vi "GetSingleAnalogInputVal.vi"(8 "error in (no error)":errorcluster, 11 "SerialPortRef":T1) -> (0 "error out":errorcluster, 1 "Scaled Voltage":dbl, 2 "Raw Voltage":u32, 3 "SerialPortRef 2":T1)   [LabVIEW 2015]
uses:
  <vilib>/Rock Robotics/WPI/SerialPort/WPI_SerialPortRef.ctl
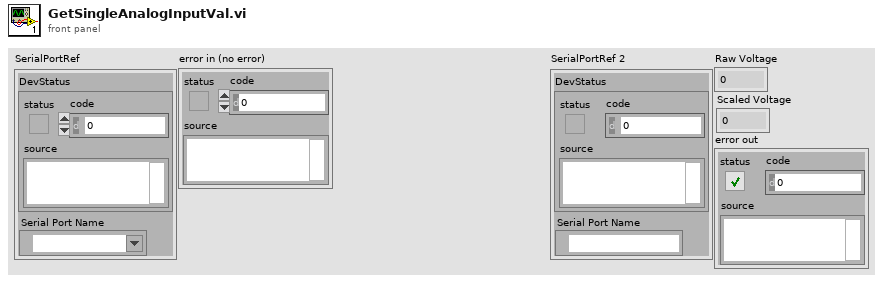
[diagram p1: front panel]
types:
  T1 = typedef "WPI_SerialPortRef.ctl" = cluster{"DevStatus":errorcluster, "Serial Port Name":refnum<visa-resource-name>}
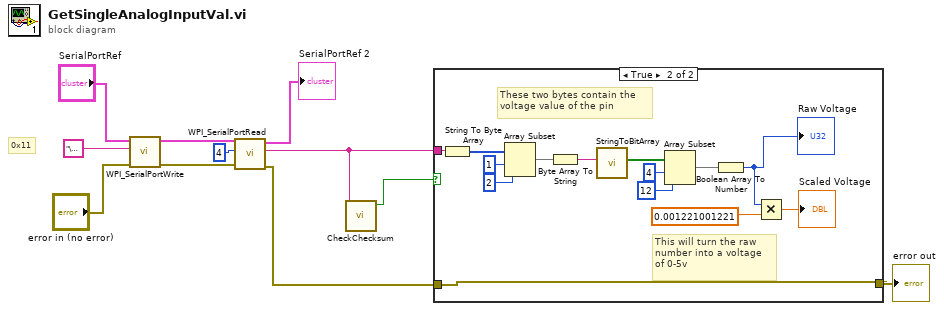
[diagram p0: block diagram]
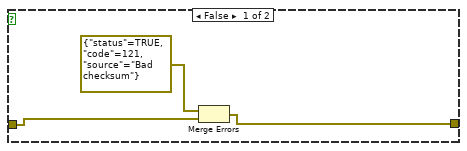
[diagram p2: hidden frame]
diagram:
  # "0x11"
  n1 = call <vilib>:"WPI_SerialPortWrite.vi"("error in (no error)"="error in (no error)", "Buffer"="\u0011", "SerialPortRef"="SerialPortRef") -> ("error out"=w7:errorcluster, "SerialPortRef"=w11:T1)  [unwired: 6 in, 1 out]
  n2 = call <vilib>:"WPI_SerialPortRead.vi"("error in (no error)"=w7, "Num Bytes to Read"=u32 4, "SerialPortRef"=w11) -> ("error out"=w1:errorcluster, "Buffer"=w4:string, "SerialPortRef"=→"SerialPortRef 2":T1)  [unwired: 6 in]
  n3 = call "CheckChecksum.vi"("String"=w4) -> ("x = y?"=w3:bool)  [unwired: 10 in]
  n4 = case shown="True" w3 {
    tunnel: w4 -> [_ w16]
    tunnel: w1 -> [w14 w15]
    tunnel: [w12 w15] -> w2
    frame False {
      n5 = Merge Errors(errorcluster {"status"=TRUE, "code"=121, "source"="Bad checksum"} ("error in"), w14) -> (w12:errorcluster)
    }
    frame True {
      # "This will turn the raw \nnumber into a voltage \nof 0-5v"
      # "These two bytes contain the \nvoltage value of the pin"
      n6 = String To Byte Array(string=w16) -> (unsigned byte array=w28:u8[])
      n7 = Array Subset(array=w28, index=1, length=2) -> (w25:u8[])
      n8 = Byte Array To String(unsigned byte array=w25) -> (string=w24:string)
      n9 = call "StringToBitArray.vi"("string"=w24) -> ("Array"=w23:bool[])  [unwired: 10 in]
      n10 = Array Subset(array=w23, index=4, length=12) -> (w20:bool[])
      n11 = Boolean Array To Number(Boolean array=w20) -> (number=w19:u32)
      "Raw Voltage" <- w19
      n12 = Multiply(x=w19, y=0.001221001221) -> (x*y=→"Scaled Voltage":dbl)
    }
  }
  "error out" <- w2
